vi "Read_current-message.vi"(8 "error in (no error)":errorcluster, 11 "Message in":refnum<class "Message.lvclass">) -> (0 "error out":errorcluster, 1 "message string":string, 2 "time string":string, 3 "Message out":refnum<class "Message.lvclass">, 4 "current message":cluster{"time string":string, "message":string})   [LabVIEW 2018, in "Message.lvclass"]
uses:
  Message.lvclass
  Message.lvclass/Message.ctl
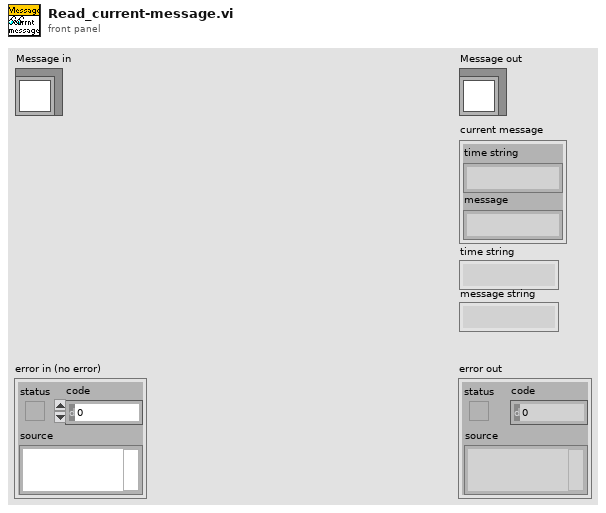
[diagram p1: front panel]
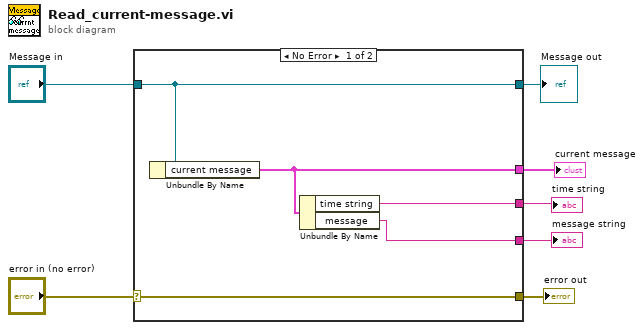
[diagram p0: block diagram]
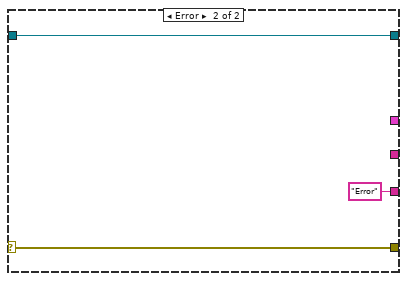
[diagram p2: hidden frame]
diagram:
  n1 = case shown="No Error" "error in (no error)" {
    selector: "error in (no error)" -> [w12 w14]
    tunnel: [w12 w14] -> w6
    tunnel: [w11 w15] -> w4
    tunnel: "Message in" -> [w11 w15]
    tunnel: [w10 _] -> w3
    tunnel: [w9 _] -> w2
    tunnel: [w8 "Error" ("message")] -> w1
    frame No Error {
      n2 = Unbundle By Name(w11) -> ("current message"=w10:cluster{"time string":string, "message":string})
      n3 = Unbundle By Name(w10) -> ("time string"=w9:string, "message"=w8:string)
    }
    frame Error {
    }
  }
  "error out" <- w6
  "Message out" <- w4
  "current message" <- w3
  "time string" <- w2
  "message string" <- w1
